vi "EnemyBallPossesion.vi"(9 "Id Duelist":u32, 10 "Atacando contra?":bool=TRUE, 11 "IA State Input":T1={"our_robots"=[], "enemy_robots"=[], "balls"=[], "geometry"={"line_width"=0, "field_length"=0, "field_width"=0, "boundary_width"=0, "referee_width"=0, "goal_width"=0, "goal_depth"=0, "goal_wall_width"=0, "center_circle_radius"=0, "defense_radius"=0, "defense_stretch"=0, "free_kick_from_defense_dist"=0, "penalty_spot_from_field_line_dist"=0, "penalty_line_from_spot_dist"=0}, "IA Judge"={"stage"="", "command"="", "our_goalie_id"=0.0, "enemy_goalie_id"=0.0, "command enum"=enum."Halt", "Time"=enum."Azul"}, "Received Timestamp"=timestamp(0 s since 1904-01-01), "Events"={"Touch"=FALSE, "Ball out"=FALSE, "id touch"=0.0, "Ball out of \nVision"=FALSE, "Ball inside \nGoalie area"=FALSE, "Robot not responding"=FALSE, "Robots responding status"=[1.0, 1.0, 1.0, 1.0, 1.0, 1.0], "Enemy Ball \nPossession"=FALSE, "Pass State"=FALSE, "id end of pass"=0.0, "Kick"=FALSE, "Id ini Possession"=0.0, "Ball Possesion"=FALSE, "Id Possesion"=0.0, "Direct Kick"=FALSE}}) -> (0 "Id Enemy Ball Possesion":u32, 3 "Enemy Ball Possesion?":bool)   [LabVIEW 2017]
uses:
  Core/AI Input.ctl
  Core/AI Robot.ctl
  Functions Enum.ctl
  AttackerStates.ctl
  Path Planning/RRT/PathDests.ctl
  Path Planning/RRT/PathDest.ctl
  Core/AI Ball.ctl
  Core/Field Size.ctl
  Core/AI Judge.ctl
  Command Enum.ctl
  Util/Events/Events.ctl
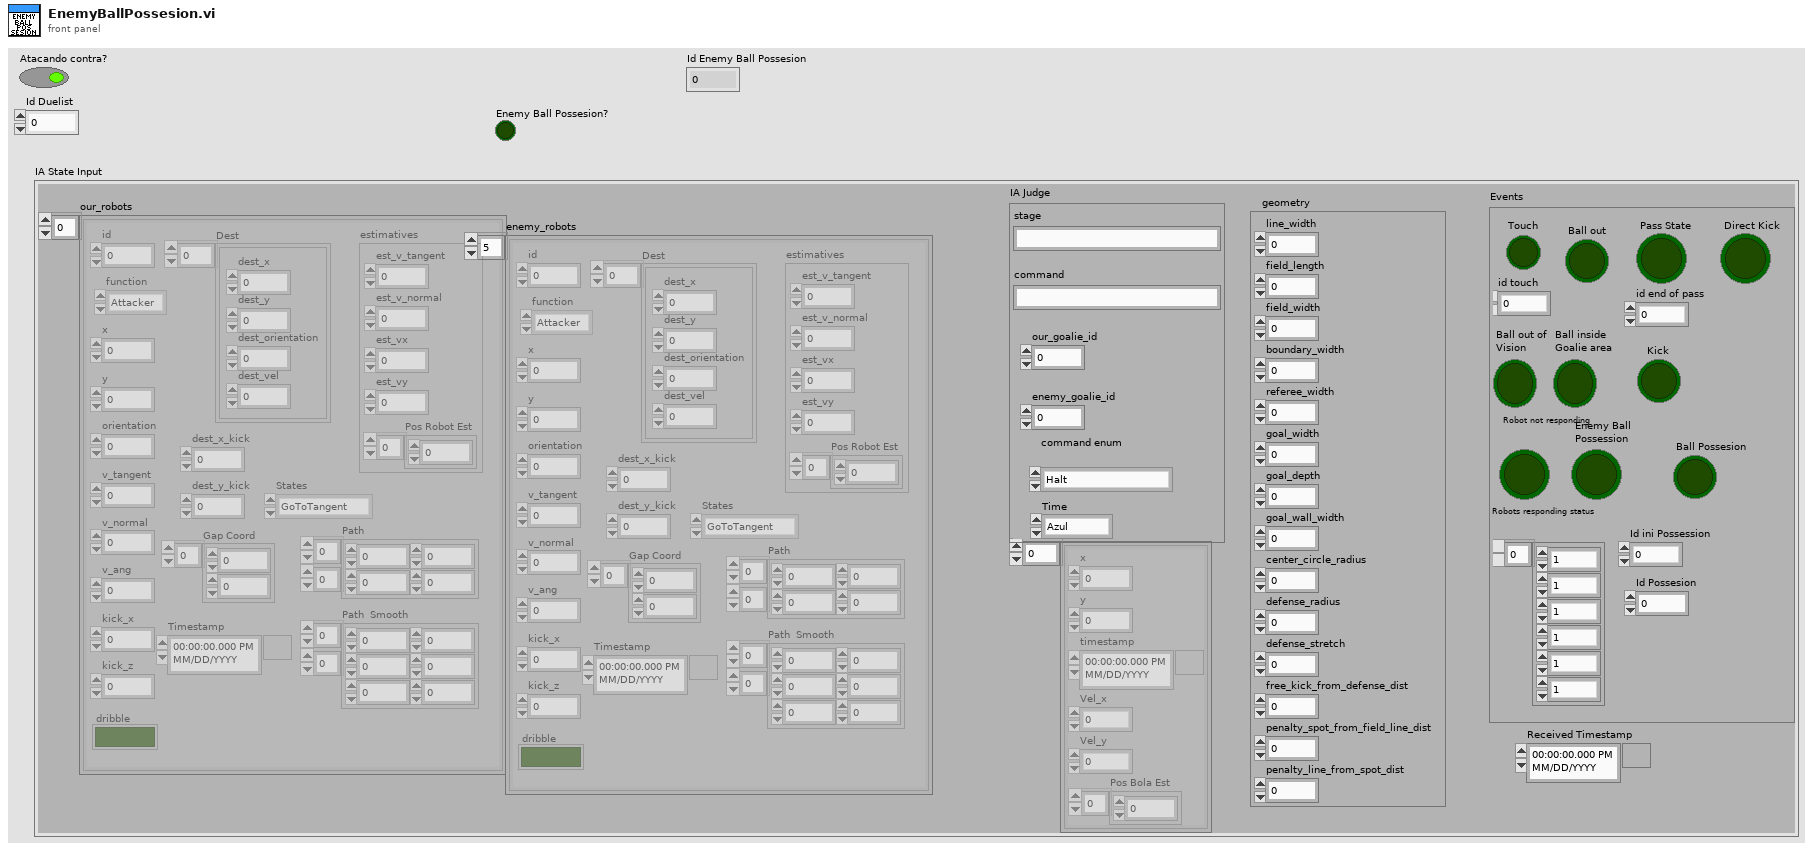
[diagram p1: front panel]
types:
  T1 = typedef "AI Input.ctl" = cluster{"our_robots":T2[], "enemy_robots":T2[], "balls":T7[], "geometry":T8, "IA Judge":T9, "Received Timestamp":timestamp, "Events":T11}
  T2 = typedef "AI Robot.ctl" = cluster{"id":u32, "function":T3, "x":dbl, "y":dbl, "orientation":dbl, "v_tangent":dbl, "v_normal":dbl, "v_ang":dbl, "kick_x":dbl, "kick_z":dbl, "dribble":bool, "Timestamp":timestamp, "estimatives":cluster{"est_v_tangent":dbl, "est_v_normal":dbl, "est_vx":dbl, "est_vy":dbl, "Pos Robot Est":dbl[]}, "dest_x_kick":dbl, "dest_y_kick":dbl, "Gap Coord":dbl[], "States":T4, "Path ":dbl[][], "Path  Smooth":dbl[][], "Dest":T5}
  T3 = typedef "Functions Enum.ctl" = enum16{"Attacker", "Goalie", "Defender", "Striker", "Goto 0", "Dummy", "Kicker", "ZigZag 0", "ZigZag 1", "ZigZag 2", "ZigZag 3", "ZigZag 4", "ZigZag 5", "ZigZag 6", "ZigZag 7", "ZigZag 8", ""}
  T4 = typedef "AttackerStates.ctl" = enum16{"Pass", "GoToTangent", "BallGetting", "GoToKick", ""}
  T5 = typedef "PathDests.ctl" = T6[]
  T6 = typedef "PathDest.ctl" = cluster{"dest_x":dbl, "dest_y":dbl, "dest_orientation":dbl, "dest_vel":dbl}
  T7 = typedef "AI Ball.ctl" = cluster{"x":dbl, "y":dbl, "timestamp":timestamp, "Vel_x":dbl, "Vel_y":dbl, "Pos Bola Est":dbl[]}
  T8 = typedef "Field Size.ctl" = cluster{"line_width":u32, "field_length":u32, "field_width":u32, "boundary_width":u32, "referee_width":u32, "goal_width":u32, "goal_depth":u32, "goal_wall_width":u32, "center_circle_radius":u32, "defense_radius":u32, "defense_stretch":u32, "free_kick_from_defense_dist":u32, "penalty_spot_from_field_line_dist":u32, "penalty_line_from_spot_dist":u32}
  T9 = typedef "AI Judge.ctl" = cluster{"stage":string, "command":string, "our_goalie_id":dbl, "enemy_goalie_id":dbl, "command enum":T10, "Time":enum16{"Azul", "Amarelo"}}
  T10 = typedef "Command Enum.ctl" = enum16{"Halt", "Stop", "Force Start", "PKA Normal Start", "Prepare Kickoff Ally", "PKE Normal Start", "Prepare Kickoff Enemy", "Prepare Penalty Ally", "PPA Normal Start", "Prepare Penalty Enemy", "PPE Normal Start", "Direct Free Enemy", "Direct Free Ally", "Indirect Free Enemy", "Indirect Free Ally", "Timeout Enemy", "Timeout Ally", "Goal Enemy", "Goal Ally", "Ball Placement Enemy", "Ball Placement Ally", "Normal Half Time", "Extra Time Break", "Extra Half Time", "None", "Post Game"}
  T11 = typedef "Events.ctl" = cluster{"Touch":bool, "Ball out":bool, "id touch":dbl, "Ball out of \nVision":bool, "Ball inside \nGoalie area":bool, "Robot not responding":bool, "Robots responding status":dbl[], "Enemy Ball \nPossession":bool, "Pass State":bool, "id end of pass":dbl, "Kick":bool, "Id ini Possession":dbl, "Ball Possesion":bool, "Id Possesion":dbl, "Direct Kick":bool}
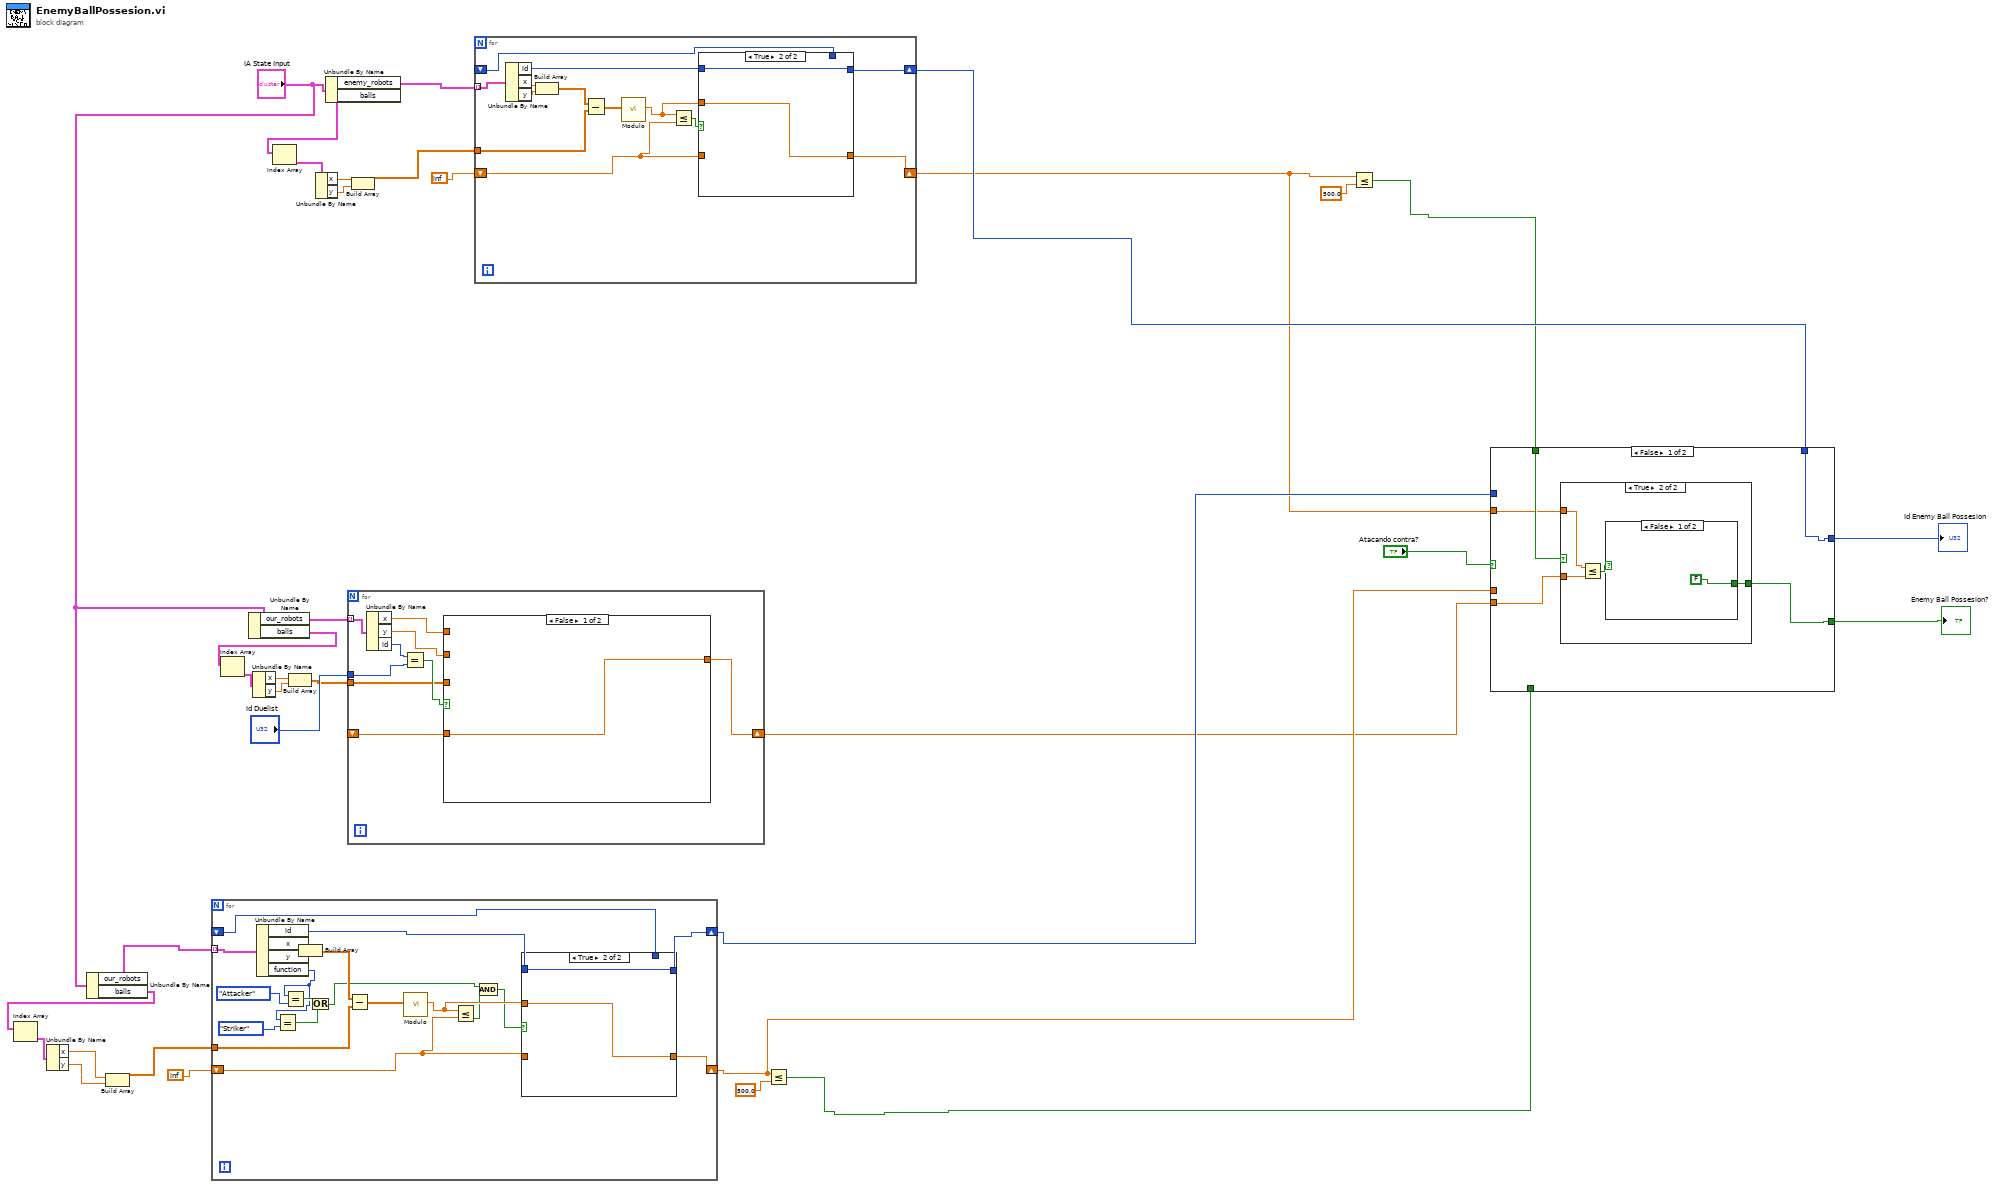
[diagram p0: block diagram]
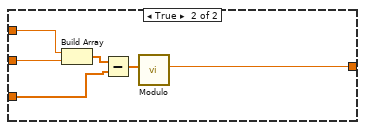
[diagram p2: hidden frame]
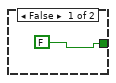
[diagram p3: hidden frame]
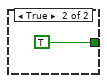
[diagram p4: hidden frame]
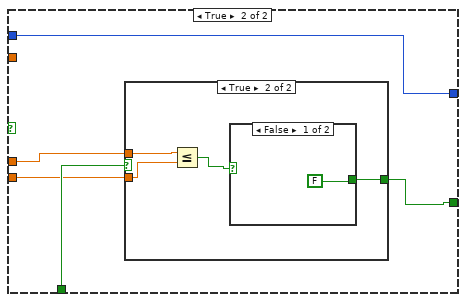
[diagram p5: hidden frame]
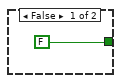
[diagram p6: hidden frame]
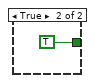
[diagram p7: hidden frame]
diagram:
  n1 = Unbundle By Name("IA State Input") -> ("our_robots"=w24:T2[], "balls"=w22:T7[])
  n2 = Index Array(array=w22) -> (element=w21:T7)  [unwired: 1 in]
  n3 = Unbundle By Name(w21) -> ("x"=w20:dbl, "y"=w19:dbl)
  n4 = Build Array(w20, w19) -> (w23:dbl[])
  n5 = for {
    tunnel: w24 -> [w54] mode=indexing
    tunnel: w23 -> [w50]
    shift-right: [w48] -> w5
    shift-left: inf -> [w46]
    shift-right: [w44] -> w15
    shift-left: _ -> [w43]
    n6 = Unbundle By Name(w54) -> ("id"=w45:u32, "x"=w53:dbl, "y"=w52:dbl, "function"=w38:T3)
    n7 = Equal?(x=w38, y=Functions_Enum."Striker" ("function")) -> (x = y?=w37:bool)
    n8 = Equal?(x=w38, y=Functions_Enum."Attacker" ("function")) -> (x = y?=w40:bool)
    n9 = Build Array(w53, w52) -> (w51:dbl[])
    n10 = Or(x=w40, y=w37) -> (x .or. y?=w36:bool)
    n11 = Subtract(x=w51, y=w50) -> (x-y=w49:dbl[])
    n12 = call "Modulo.vi"("2D vector"=w49) -> ("Modulo"=w47:dbl)  [unwired: 10 in]
    n13 = Less Or Equal?(x=w47, y=w46) -> (x <= y?=w42:bool)
    n14 = And(x=w36, y=w42) -> (x .and. y?=w35:bool)
    n15 = case shown="True" w35 {
      tunnel: [w56 w58] -> w48
      tunnel: w47 -> [_ w58]
      tunnel: w46 -> [w56 _]
      tunnel: [w55 w57] -> w44
      tunnel: w45 -> [_ w57]
      tunnel: w43 -> [w55 _]
      frame False {
      }
      frame True {
      }
    }
  }
  n16 = Unbundle By Name("IA State Input") -> ("our_robots"=w12:T2[], "balls"=w10:T7[])
  n17 = Index Array(array=w10) -> (element=w9:T7)  [unwired: 1 in]
  n18 = Unbundle By Name(w9) -> ("x"=w8:dbl, "y"=w7:dbl)
  n19 = Build Array(w8, w7) -> (w6:dbl[])
  n20 = Unbundle By Name("IA State Input") -> ("enemy_robots"=w28:T2[], "balls"=w34:T7[])
  n21 = Index Array(array=w34) -> (element=w33:T7)  [unwired: 1 in]
  n22 = Unbundle By Name(w33) -> ("x"=w32:dbl, "y"=w31:dbl)
  n23 = for {
    tunnel: w12 -> [w67] mode=indexing
    tunnel: "Id Duelist" -> [w65]
    tunnel: w6 -> [w61]
    shift-right: [w60] -> w4
    shift-left: _ -> [w59]
    n24 = Unbundle By Name(w67) -> ("x"=w63:dbl, "y"=w62:dbl, "id"=w66:u32)
    n25 = Equal?(x=w66, y=w65) -> (x = y?=w64:bool)
    n26 = case shown="False" w64 {
      tunnel: w63 -> [_ w74]
      tunnel: w62 -> [_ w73]
      tunnel: w61 -> [_ w71]
      tunnel: [w68 w69] -> w60
      tunnel: w59 -> [w68 _]
      frame False {
      }
      frame True {
        n27 = Build Array(w74, w73) -> (w72:dbl[])
        n28 = Subtract(x=w72, y=w71) -> (x-y=w70:dbl[])
        n29 = call "Modulo.vi"("2D vector"=w70) -> ("Modulo"=w69:dbl)  [unwired: 10 in]
      }
    }
  }
  n30 = Build Array(w32, w31) -> (w27:dbl[])
  n31 = for {
    tunnel: w28 -> [w87] mode=indexing
    tunnel: w27 -> [w83]
    shift-right: [w80] -> w1
    shift-left: inf -> [w78]
    shift-right: [w76] -> w14
    shift-left: _ -> [w75]
    n32 = Unbundle By Name(w87) -> ("id"=w77:u32, "x"=w86:dbl, "y"=w85:dbl)
    n33 = Build Array(w86, w85) -> (w84:dbl[])
    n34 = Subtract(x=w84, y=w83) -> (x-y=w82:dbl[])
    n35 = call "Modulo.vi"("2D vector"=w82) -> ("Modulo"=w79:dbl)  [unwired: 10 in]
    n36 = Less Or Equal?(x=w79, y=w78) -> (x <= y?=w81:bool)
    n37 = case shown="True" w81 {
      tunnel: [w89 w91] -> w80
      tunnel: w79 -> [_ w91]
      tunnel: w78 -> [w89 _]
      tunnel: [w88 w90] -> w76
      tunnel: w77 -> [_ w90]
      tunnel: w75 -> [w88 _]
      frame False {
      }
      frame True {
      }
    }
  }
  n38 = Less Or Equal?(x=w5, y=500.0) -> (x <= y?=w3:bool)
  n39 = Less Or Equal?(x=w1, y=500.0) -> (x <= y?=w2:bool)
  n40 = case shown="False" "Atacando contra?" {
    tunnel: [w92 w104] -> w17
    tunnel: [w96 w108] -> w16
    tunnel: w15 -> [_ w108]
    tunnel: w14 -> [w96 _]
    tunnel: w5 -> [_ w106]
    tunnel: w4 -> [w94 w105]
    tunnel: w3 -> [_ w107]
    tunnel: w2 -> [w95 _]
    tunnel: w1 -> [w93 _]
    frame False {
      n41 = case shown="True" w95 {
        tunnel: w94 -> [_ w101]
        tunnel: w93 -> [_ w100]
        tunnel: [FALSE w98] -> w92
        frame False {
        }
        frame True {
          n42 = Less Or Equal?(x=w100, y=w101) -> (x <= y?=w99:bool)
          n43 = case shown="False" w99 {
            tunnel: [FALSE TRUE] -> w98
            frame False {
            }
            frame True {
            }
          }
        }
      }
    }
    frame True {
      n44 = case shown="True" w107 {
        tunnel: w106 -> [_ w113]
        tunnel: w105 -> [_ w112]
        tunnel: [FALSE w110] -> w104
        frame False {
        }
        frame True {
          n45 = Less Or Equal?(x=w113, y=w112) -> (x <= y?=w111:bool)
          n46 = case shown="False" w111 {
            tunnel: [FALSE TRUE] -> w110
            frame False {
            }
            frame True {
            }
          }
        }
      }
    }
  }
  "Enemy Ball Possesion?" <- w17
  "Id Enemy Ball Possesion" <- w16
